vi "IDLE.vi"(11 "Class 2.lvclass":refnum<class "Class 2.lvclass">) -> (3 "Class 2.lvclass 2":refnum<class "Class 2.lvclass">)   [LabVIEW 2019, in "Class 2.lvclass"]
uses:
  Class 2.lvclass
  Class 2.lvclass/Class 2.ctl
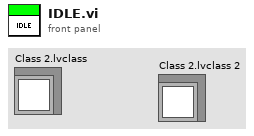
[diagram p1: front panel]
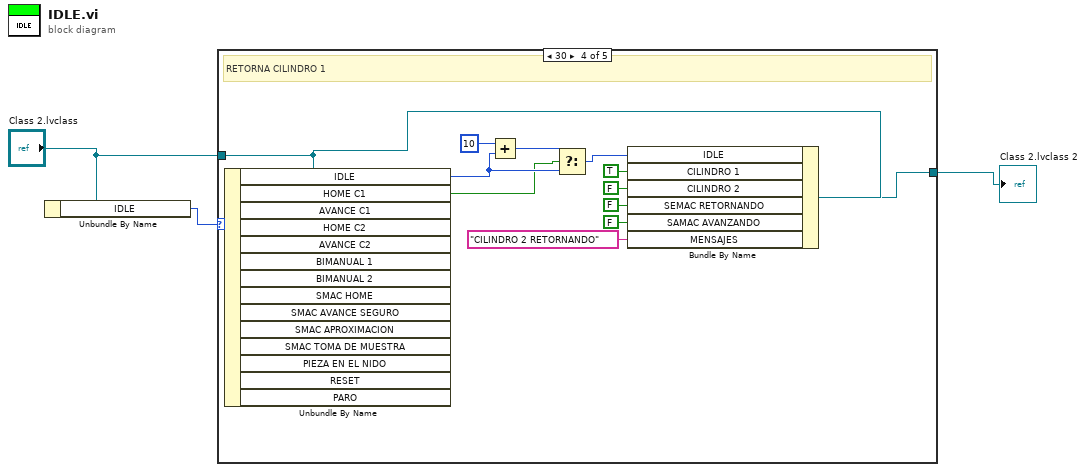
[diagram p0: block diagram]
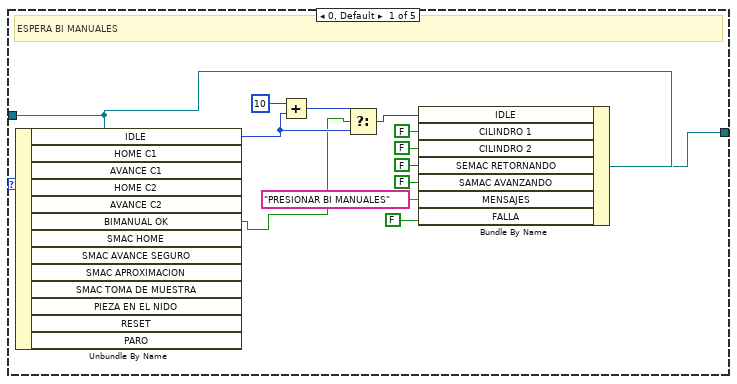
[diagram p2: hidden frame]
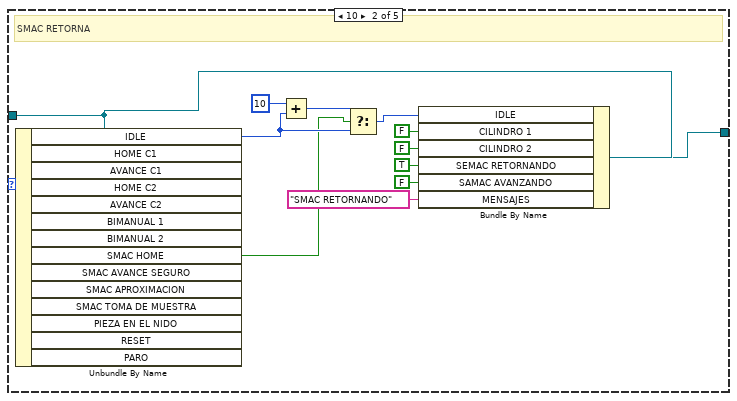
[diagram p3: hidden frame]
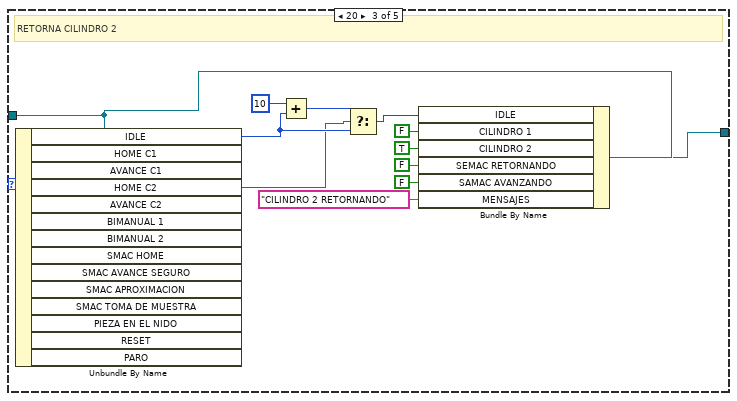
[diagram p4: hidden frame]
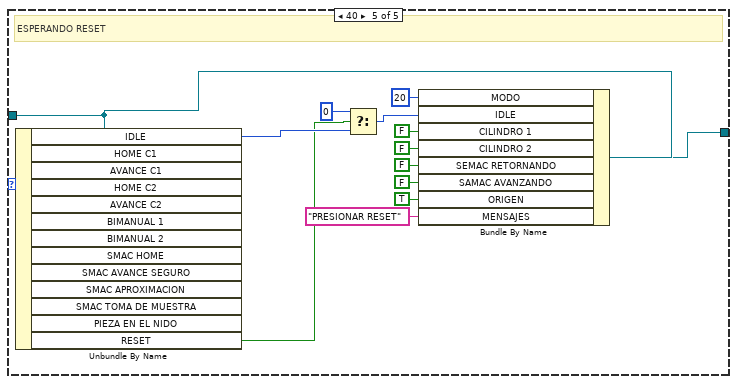
[diagram p5: hidden frame]
diagram:
  n1 = Unbundle By Name("Class 2.lvclass") -> ("IDLE"=w3:i16)
  n2 = case shown="30" w3 {
    tunnel: "Class 2.lvclass" -> [w15 w27 w39 w51 w65]
    tunnel: [w14 w26 w38 w50 w64] -> w1
    frame 0, Default {
      # "ESPERA BI MANUALES"
      n3 = Unbundle By Name(w15) -> ("IDLE"=w11:i16, "BIMANUAL OK"=w4:bool)  [unwired: 11 out]
      n4 = Add(x=i16 10, y=w11) -> (x+y=w13:i16)
      n5 = Select(t=w13, s=w4, f=w11) -> (s? t:f=w12:i16)
      n6 = Bundle By Name(cluster=w15, "IDLE"=w12, "CILINDRO 1"=FALSE ("SALIDAS.CILINDRO 1"), "CILINDRO 2"=FALSE ("SALIDAS.CILINDRO 2"), "SEMAC RETORNANDO"=FALSE ("SALIDAS.SEMAC RETORNANDO"), "SAMAC AVANZANDO"=FALSE ("SALIDAS.SAMAC AVANZANDO"), "MENSAJES"="PRESIONAR BI MANUALES" ("SALIDAS.MENSAJES"), "FALLA"=FALSE ("PROCESO.FALLA")) -> (w14:refnum<class "Class 2.lvclass">)
    }
    frame 10 {
      # "SMAC RETORNA"
      n7 = Unbundle By Name(w27) -> ("IDLE"=w23:i16, "SMAC HOME"=w18:bool)  [unwired: 12 out]
      n8 = Add(x=i16 10, y=w23) -> (x+y=w25:i16)
      n9 = Select(t=w25, s=w18, f=w23) -> (s? t:f=w24:i16)
      n10 = Bundle By Name(cluster=w27, "IDLE"=w24, "CILINDRO 1"=FALSE ("SALIDAS.CILINDRO 1"), "CILINDRO 2"=FALSE ("SALIDAS.CILINDRO 2"), "SEMAC RETORNANDO"=TRUE ("SALIDAS.SEMAC RETORNANDO"), "SAMAC AVANZANDO"=FALSE ("SALIDAS.SAMAC AVANZANDO"), "MENSAJES"="SMAC RETORNANDO" ("SALIDAS.MENSAJES")) -> (w26:refnum<class "Class 2.lvclass">)
    }
    frame 20 {
      # "RETORNA CILINDRO 2"
      n11 = Unbundle By Name(w39) -> ("IDLE"=w35:i16, "HOME C2"=w30:bool)  [unwired: 12 out]
      n12 = Add(x=i16 10, y=w35) -> (x+y=w37:i16)
      n13 = Select(t=w37, s=w30, f=w35) -> (s? t:f=w36:i16)
      n14 = Bundle By Name(cluster=w39, "IDLE"=w36, "CILINDRO 1"=FALSE ("SALIDAS.CILINDRO 1"), "CILINDRO 2"=TRUE ("SALIDAS.CILINDRO 2"), "SEMAC RETORNANDO"=FALSE ("SALIDAS.SEMAC RETORNANDO"), "SAMAC AVANZANDO"=FALSE ("SALIDAS.SAMAC AVANZANDO"), "MENSAJES"="CILINDRO 2 RETORNANDO" ("SALIDAS.MENSAJES")) -> (w38:refnum<class "Class 2.lvclass">)
    }
    frame 30 {
      # "RETORNA CILINDRO 1"
      n15 = Unbundle By Name(w51) -> ("IDLE"=w47:i16, "HOME C1"=w42:bool)  [unwired: 12 out]
      n16 = Add(x=i16 10, y=w47) -> (x+y=w49:i16)
      n17 = Select(t=w49, s=w42, f=w47) -> (s? t:f=w48:i16)
      n18 = Bundle By Name(cluster=w51, "IDLE"=w48, "CILINDRO 1"=TRUE ("SALIDAS.CILINDRO 1"), "CILINDRO 2"=FALSE ("SALIDAS.CILINDRO 2"), "SEMAC RETORNANDO"=FALSE ("SALIDAS.SEMAC RETORNANDO"), "SAMAC AVANZANDO"=FALSE ("SALIDAS.SAMAC AVANZANDO"), "MENSAJES"="CILINDRO 2 RETORNANDO" ("SALIDAS.MENSAJES")) -> (w50:refnum<class "Class 2.lvclass">)
    }
    frame 40 {
      # "ESPERANDO RESET"
      n19 = Unbundle By Name(w65) -> ("IDLE"=w63:i16, "RESET"=w58:bool)  [unwired: 11 out]
      n20 = Select(t=i16 0, s=w58, f=w63) -> (s? t:f=w55:i16)
      n21 = Bundle By Name(cluster=w65, "MODO"=i16 20 ("MAQ DE ESTADOS.MODO"), "IDLE"=w55, "CILINDRO 1"=FALSE ("SALIDAS.CILINDRO 1"), "CILINDRO 2"=FALSE ("SALIDAS.CILINDRO 2"), "SEMAC RETORNANDO"=FALSE ("SALIDAS.SEMAC RETORNANDO"), "SAMAC AVANZANDO"=FALSE ("SALIDAS.SAMAC AVANZANDO"), "ORIGEN"=TRUE ("PROCESO.ORIGEN"), "MENSAJES"="PRESIONAR RESET" ("SALIDAS.MENSAJES")) -> (w64:refnum<class "Class 2.lvclass">)
    }
  }
  "Class 2.lvclass 2" <- w1
